vi "Get Settings.vi"(8 "error in (no error)":errorcluster, 11 "Component Settings Editor in":refnum<class "Component Settings Editor.lvclass">) -> (0 "error out":errorcluster, 2 "component settings":T1[](array[typedef]), 3 "Component Settings Editor out":refnum<class "Component Settings Editor.lvclass">)   [LabVIEW 2019, in "DSF Core.lvlib" / "Component Settings Editor.lvclass"]
uses:
  Component Settings Editor.lvclass
  Typedefs/DSF Settings Info.ctl
  Component Settings Editor.lvclass/Component Settings Editor.ctl
  User Interface.lvclass
  DSF Core.lvlib
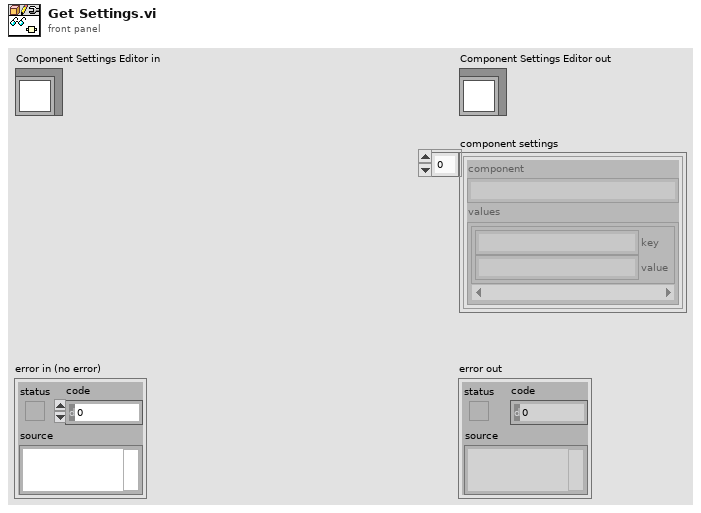
[diagram p1: front panel]
types:
  T1 = typedef "DSF Core.lvlib/DSF Settings Info.ctl" = cluster{"component":string, "values":cluster{"key":string, "value":string}[]}
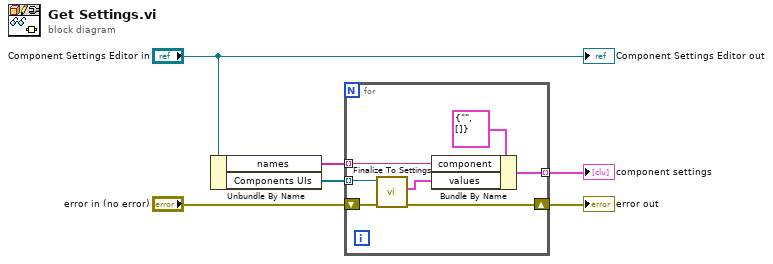
[diagram p0: block diagram]
diagram:
  n1 = Unbundle By Name("Component Settings Editor in") -> ("names"=w5:string[], "Components UIs"=w4:refnum<class "User Interface.lvclass">[])
  n2 = for {
    tunnel: w5 -> [w11] mode=indexing
    tunnel: w4 -> [w13] mode=indexing
    tunnel: [w9] -> w3 mode=indexing
    shift-right: [w7] -> w2
    shift-left: "error in (no error)" -> [w8]
    n3 = call "Finalize To Settings.vi"("error in (no error)"=w8, "User Interface in"=w13) -> ("error out"=w7:errorcluster, "settings"=w10:cluster{"key":string, "value":string}[])  [unwired: 7 in, 1 out]
    n4 = Bundle By Name(cluster=T1 {"component"="", "values"=[]} ("component settings"), "component"=w11, "values"=w10) -> (w9:T1)
  }
  "error out" <- w2
  "component settings" <- w3
  "Component Settings Editor out" <- "Component Settings Editor in"
